vi "setClockChans.vi"(0 "Analogue Data (volts)":dbl[][](array[numeric])) -> (1 "LSB":dbl[](array[numeric]), 2 "MSB":dbl[](array[numeric]))   [LabVIEW 2017]
uses:
  Controls/chanType.ctl
  Globals/measurementGlobal.vi
panel:
  out "MSB":dbl[](graph)
  out "LSB":dbl[](graph)
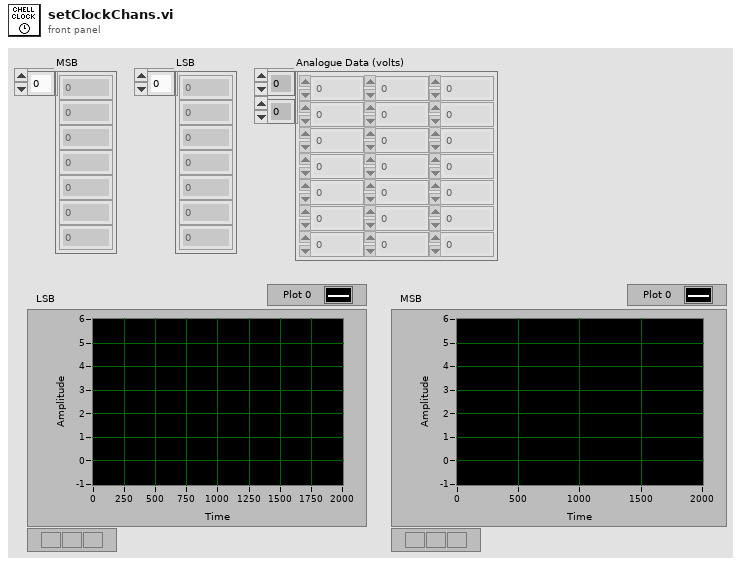
[diagram p1: front panel]
types:
  T1 = cluster{"Most Significant Bit":dbl, "Least Significant Bit":dbl}[]
  T2 = typedef "chanType.ctl" = enum16{"Default", "Clock", "Pressure Scanner"}
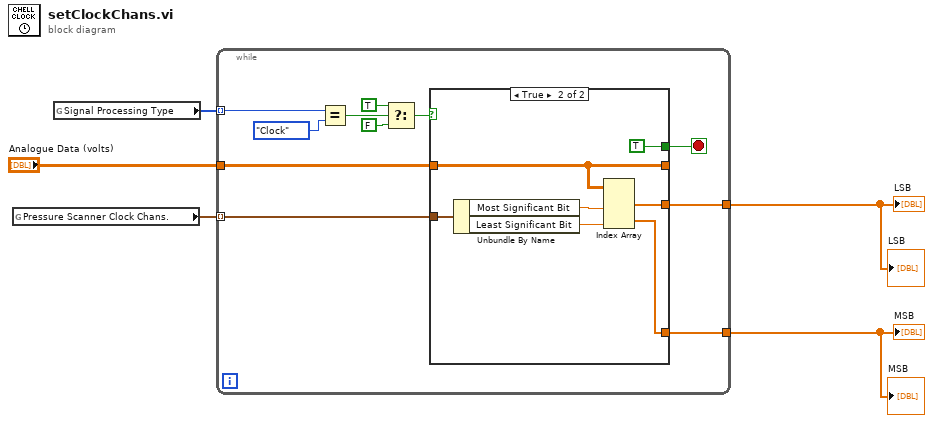
[diagram p0: block diagram]
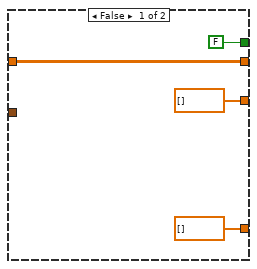
[diagram p2: hidden frame]
diagram:
  n1 = global read "measurementGlobal.vi" "Pressure Scanner Clock Chans."() -> (w5:T1)
  n2 = global read "measurementGlobal.vi" "Signal Processing Type"() -> (w2:T2[])
  n3 = while {
    tunnel: "Analogue Data (volts)" -> [w14]
    tunnel: w5 -> [w16] mode=indexing
    tunnel: [w13] -> w4
    tunnel: [w15] -> w3
    tunnel: w2 -> [w7] mode=indexing
    stop <- w8 stop-if-true
    n4 = Equal?(x=w7, y=chanType."Clock") -> (x = y?=w12:bool)
    n5 = Select(t=TRUE, s=w12, f=FALSE) -> (s? t:f=w9:bool)
    n6 = case shown="True" w9 {
      tunnel: w16 -> [_ w27]
      tunnel: [dbl[] [] ("Analogue Data (volts)") w26] -> w15
      tunnel: w14 -> [w20 w21]
      tunnel: [w20 w21] -> _
      tunnel: [dbl[] [] ("Analogue Data (volts)") w23] -> w13
      tunnel: [FALSE TRUE] -> w8
      frame False {
      }
      frame True {
        n7 = Unbundle By Name(w27) -> ("Most Significant Bit"=w25:dbl, "Least Significant Bit"=w24:dbl)
        n8 = Index Array(array=w21, index (col) #1=w25, index (col) #2=w24) -> (element #1=w23:dbl[], element #2=w26:dbl[])  [unwired: 2 in]
      }
    }
  }
  "LSB" <- w4
  "MSB" <- w3
  "LSB" <- w4
  "MSB" <- w3
